vi "Omega start.vi"() -> ()   [LabVIEW 2019]
doc: "Thus VI communicates with \"alpha\" via the collection of global variables in \"tau\".\n\nIt can clear the global.\n\nIt stops automatically under \"alpha\" command.\n\nJuan Gamez\nP3600\nCSUSB Physics"
uses:
  globals/Tau start.vi
panel:
  out "Active":bool
  in  "publish info":bool
  out "text read from global":string
  out "number read from global":dbl
  in  "text to publish":string="Hello Alpha"
  in  "number to publish":dbl=7.0
  in  "grab info":bool
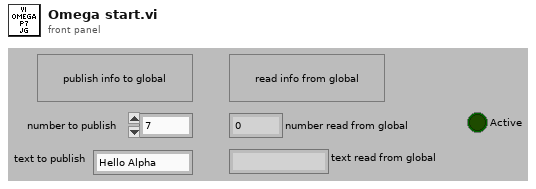
[diagram p1: front panel]
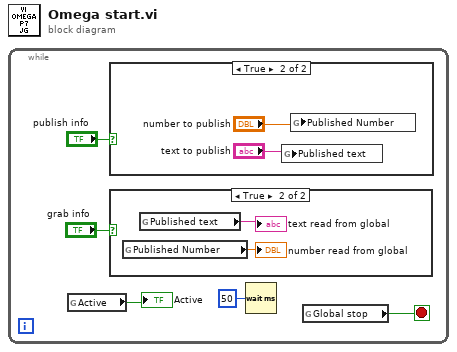
[diagram p0: block diagram]
diagram:
  n1 = while {
    stop <- w2 stop-if-true
    n2 = global read "Tau start.vi" "Active"() -> (→"Active":bool)
    n3 = case shown="True" "publish info" {
      frame False {
      }
      frame True {
        n4 = global write "Tau start.vi" "Published text"("text to publish") -> ()
        n5 = global write "Tau start.vi" "Published Number"("number to publish") -> ()
      }
    }
    n6 = case shown="True" "grab info" {
      frame False {
      }
      frame True {
        n7 = global read "Tau start.vi" "Published Number"() -> (→"number read from global":dbl)
        n8 = global read "Tau start.vi" "Published text"() -> (→"text read from global":string)
      }
    }
    n9 = Wait (ms)(milliseconds to wait=u32 50) -> ()  [unwired: 1 out]
    n10 = global read "Tau start.vi" "Global stop"() -> (w2:bool)
  }
